vi "Stop.vi"(8 "Error In":errorcluster, 11 "reference in":refnum<class "Thermometer Multichannel.lvclass">) -> (0 "Error Out":errorcluster, 3 "reference out":refnum<class "Thermometer Multichannel.lvclass">)   [LabVIEW 2024, in "Thermometer Multichannel.lvclass"]
uses:
  Thermometer Multichannel.lvclass
  Thermometer Multichannel.lvclass/Thermometer Multichannel.ctl
  Interfaces/IRunnable/IRunnable.lvclass
  <vilib>/ActorFramework/Stop Msg/Stop Msg.lvclass
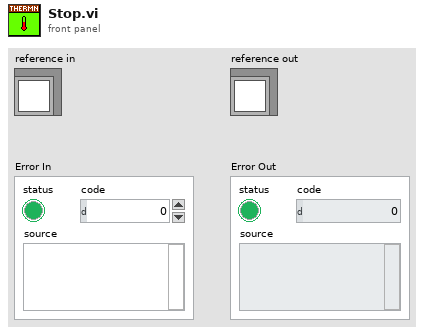
[diagram p1: front panel]
types:
  T1 = typedef "Thermometer Multichannel.lvclass/ObjectAttributes.ctl" = cluster{"IConfigure":refnum<class "IConfigure.lvclass">, "Worker Enqueuer":refnum<class "Message Enqueuer.lvclass">}
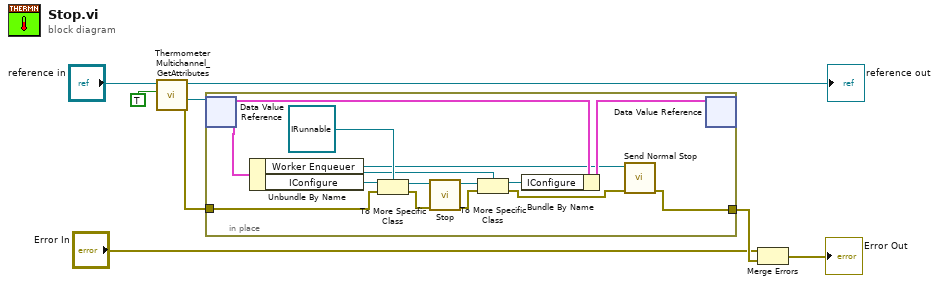
[diagram p0: block diagram]
diagram:
  n1 = call "Thermometer Multichannel_GetAttributes.vi"("OnlyGetDvrReference(False)"=TRUE, "reference in"="reference in") -> ("Error Out"=w3:errorcluster, "DataRef"=w4:refnum<data-value>, "reference out"=→"reference out":refnum<class "Thermometer Multichannel.lvclass">)  [unwired: 6 in, 1 out]
  n2 = in-place {
    in-place-border: [w9] -> w8
    in-place-border: w3 -> [w12]
    n3 = in-place-dvr #1(w4) -> (w20:T1)  [unwired: 1 out]
    n4 = Unbundle By Name(w20) -> ("Worker Enqueuer"=w11:refnum<class "Message Enqueuer.lvclass">, "IConfigure"=w13:refnum<class "IConfigure.lvclass">)
    n5 = To More Specific Class(target class=refnum<class "IRunnable.lvclass"> refnum ("IRunnable.lvclass"), reference=w13, error in=w12) -> (specific class reference=w16:refnum<class "IRunnable.lvclass">, error out=w17:errorcluster)
    n6 = call-dynamic "Stop.vi"("error in"=w17, "IRunnable in"=w16) -> ("error out"=w15:errorcluster, "IRunnable out"=w14:refnum<class "IRunnable.lvclass">)  [unwired: 8 in]
    n7 = To More Specific Class(target class=w13, reference=w14, error in=w15) -> (specific class reference=w18:refnum<class "IConfigure.lvclass">, error out=w10:errorcluster)
    n8 = Bundle By Name(cluster=w20, "IConfigure"=w18) -> (w21:T1)
    n9 = call <vilib>:"Send Normal Stop.vi"("error in (no error)"=w10, "Message Enqueuer"=w11) -> ("error out"=w9:errorcluster)  [unwired: 9 in]
    n10 = in-place-dvr #1(w21) -> ()  [unwired: 2 out]
  }
  n11 = Merge Errors("Error In", w8) -> (→"Error Out":errorcluster)
